vi "main.vi"() -> ()   [LabVIEW 2017]
uses:
  <vilib>/Utility/file.llb/Write Delimited Spreadsheet (DBL).vi
panel:
  out "saved2path":path
  out "data: time (ms), trigger, fxi, fyi, fzi, xi, yi, zi":dbl[][](array[numeric])
  in  "resample dt (s)":dbl=0.004 format="%#_13g"
  in  "marker count":i32=14
  in  "file path":path
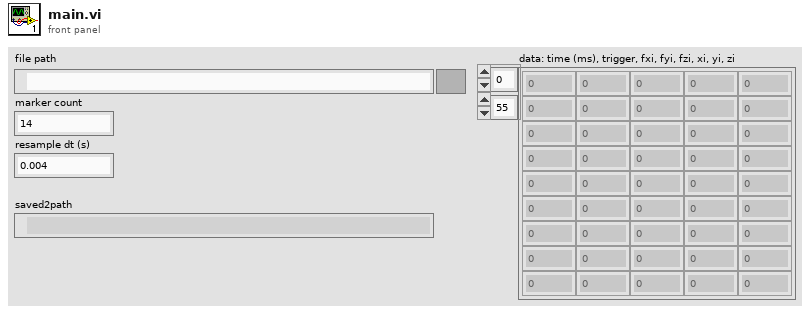
[diagram p1: front panel]
types:
  T1 = enum16{"open", "open or create", "create or replace", "create", "open (read-only)"}
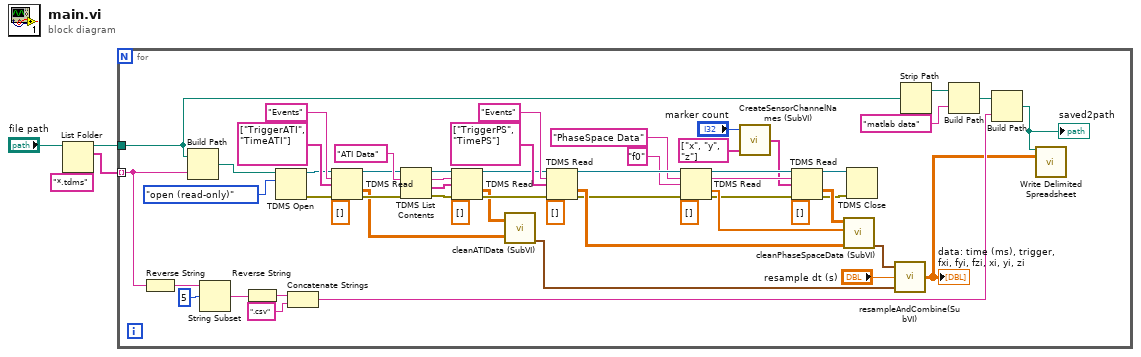
[diagram p0: block diagram]
diagram:
  n1 = List Folder(path="file path", pattern="*.tdms") -> (path out=w1:path, filenames=w2:string[])  [unwired: 2 in, 2 out]
  n2 = for {
    tunnel: w2 -> [w17] mode=indexing
    tunnel: w1 -> [w10]
    n3 = Reverse String(1:w17) -> (0:w16:string)
    n4 = Build Path(base path=w10, name or relative path=w17) -> (appended path=w18:path)
    n5 = String Subset(string=w16, offset (0)=5) -> (substring=w14:string)  [unwired: 1 in]
    n6 = Reverse String(1:w14) -> (0:w13:string)
    n7 = TDMS Open(10:T1."open (read-only)" ("operation (0:open)"), 11:w18) -> (0:w59:errorcluster, 3:w35:refnum<k34>)  [unwired: 5 in]
    n8 = Concatenate Strings(w13, ".csv") -> (w11:string)
    n9 = TDMS Read(0:w35, 5:"Events" ("group name in"), 7:string[] ["TriggerATI", "TimeATI"], 11:w59, 12:dbl[][] []) -> (4:w33:refnum<k34>, 10:w23:dbl[][], 15:w32:errorcluster)  [unwired: 3 in, 3 out]
    n10 = TDMS List Contents(4:w32, 6:"ATI Data" ("group name"), 7:w33) -> (0:w28:errorcluster, 1:w29:string[], 2:w30:string, 3:w31:refnum<k34>)
    n11 = TDMS Read(0:w31, 5:w30, 7:w29, 11:w28, 12:dbl[][] []) -> (4:w26:refnum<k34>, 10:w24:dbl[][], 15:w25:errorcluster)  [unwired: 3 in, 3 out]
    n12 = call "cleanATIData (SubVI).vi"("raw data"=w24, "raw trigger"=w23) -> ("data"=w21:waveform(dbl)[])  [unwired: 3 out]
    n13 = TDMS Read(0:w26, 5:"Events" ("group name in"), 7:string[] ["TriggerPS", "TimePS"], 11:w25, 12:dbl[][] []) -> (4:w56:refnum<k34>, 10:w41:dbl[][], 15:w38:errorcluster)  [unwired: 3 in, 3 out]
    n14 = TDMS Read(0:w56, 5:"PhaseSpace Data" ("group name in"), 7:"f0", 11:w38, 12:dbl[] []) -> (4:w53:refnum<k34>, 6:w48:string, 10:w42:dbl[], 15:w37:errorcluster)  [unwired: 3 in, 2 out]
    n15 = call "CreateSensorChannelNames (SubVI).vi"("channel name"=string[] ["x", "y", "z"], "sensor count (default: 14)"="marker count") -> ("channel names"=w45:string[])  [unwired: 3 in]
    n16 = TDMS Read(0:w53, 5:w48, 7:w45, 11:w37, 12:dbl[][] []) -> (4:w49:refnum<k34>, 10:w43:dbl[][], 15:w19:errorcluster)  [unwired: 3 in, 3 out]
    n17 = call "cleanPhaseSpaceData (SubVI).vi"("raw trigger"=w41, "raw time"=w42, "raw data"=w43) -> ("data"=w22:waveform(dbl)[])  [unwired: 1 in, 4 out]
    n18 = TDMS Close(8:w19, 11:w49) -> ()  [unwired: 2 out]
    n19 = call "resampleAndCombine(SubVI).vi"("ATI data"=w21, "resample dt (s)"="resample dt (s)", "PS data"=w22) -> ("all Data"=w5:dbl[][])  [unwired: 2 in]
    "data: time (ms), trigger, fxi, fyi, fzi, xi, yi, zi" <- w5
    n20 = Strip Path(path=w10) -> (stripped path=w8:path)  [unwired: 1 out]
    n21 = Build Path(base path=w8, name or relative path="matlab data") -> (appended path=w7:path)
    n22 = Build Path(base path=w7, name or relative path=w11) -> (appended path=w6:path)
    "saved2path" <- w6
    n23 = call-poly <vilib>:"Write Delimited Spreadsheet.vi"("file path (dialog if empty)"=w6, "2D data"=w5) -> ()  [unwired: 12 in, 2 out]
  }
